vi "Update Display.vi"(6 "Priority Message? (F)":bool, 8 "error in":errorcluster, 11 "Message string":string) -> (0 "error out":errorcluster)   [LabVIEW 2015]
uses:
  Message Queue/Message Queue.lvlib
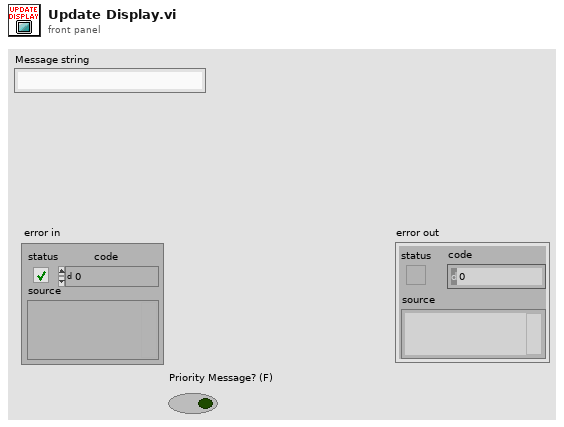
[diagram p1: front panel]
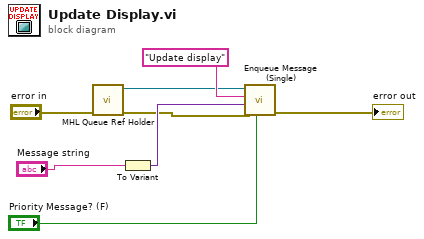
[diagram p0: block diagram]
diagram:
  n1 = call "MHL Queue Ref Holder.vi"("error in"="error in") -> ("Input Message Queue"=w1:refnum<queue>, "error out"=w2:errorcluster)  [unwired: 8 in]
  n2 = To Variant(anything="Message string") -> (Variant=w5:variant)
  n3 = call "Enqueue Message (Single).vi"("Priority Message? (F)"="Priority Message? (F)", "error in (no error)"=w2, "Message Data"=w5, "Message"="Update display", "Message Queue"=w1) -> ("error out"=→"error out":errorcluster)  [unwired: 5 in, 1 out]
